vi "NF WF1973_74 PULS Stat.vi"(8 "error in (no error)":errorcluster caption="Error IN", 9 "State(Start)":u16(ring) items=["Start", "Stop"], 10 "Ch(Ch1)":bool, 11 "VISAsession":refnum<visa-resource-name>) -> (0 "error out":errorcluster caption="Error OUT", 3 "CopyVISAsession":refnum<visa-resource-name>)   [LabVIEW 2010]
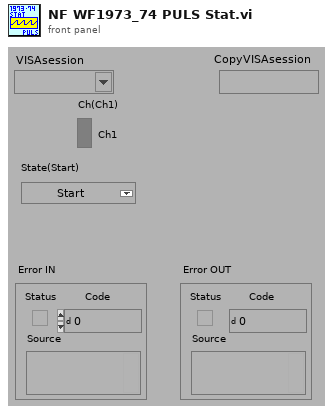
[diagram p1: front panel]
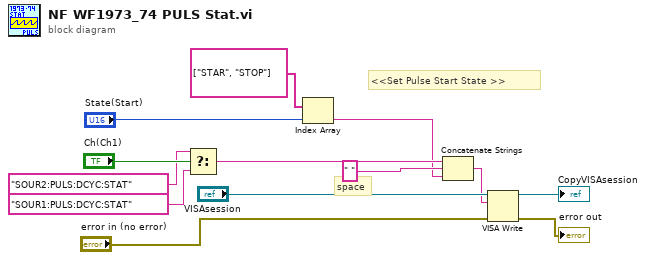
[diagram p0: block diagram]
diagram:
  # "space"
  # "<<Set Pulse Start State >>"
  n1 = Select(t="SOUR2:PULS:DCYC:STAT" ("文字列"), s="Ch(Ch1)", f="SOUR1:PULS:DCYC:STAT" ("文字列")) -> (s? t:f=w8:string)
  n2 = Index Array(array=string[] ["STAR", "STOP"], index="State(Start)") -> (element=w1:string)
  n3 = Concatenate Strings(w8, " ", w1) -> (w5:string)
  n4 = VISA Write(VISA resource name="VISAsession", write buffer=w5, error in (no error)="error in (no error)") -> (VISA resource name out=→"CopyVISAsession":refnum<visa-resource-name>, error out=→"error out":errorcluster)  [unwired: 1 out]
